vi "SW_Load_settings_to_main_tab_4.vi"(0 "Settings path in":path, 2 "Researcher name":string="Researcher", 3 "error in (no error)":errorcluster) -> (6 "Settings cluster out":T1={"Defaults"={"Default User"=0.0, "VISA Resource Name "="", "Histogram parameters"={"max"=300.0, "min"=0.0, "# bins"=10, "threshold"=8.0, "thr. type"=enum."higher accepted"}}, "Recording and saving"={"Researcher name"="", "Name prefix"="", "Data post-processing"={"Filter type"=enum."Savitzky-Golay", "Length"=31, "Order"=3}, "Stop at"=0.0, "\"Stop at\" enabled"=FALSE, "Default save folder path"=path "", "Acquisition FPS"=enum."Max"}, "Geometry"={"Sensor board size"=enum."", "Bridge swap"=FALSE, "Twisted neck"=FALSE, "Bridge H. offset"=0.0, "Bridge V. offset"=0.0, "Magnets orientation"=0.0, "Cage type"=0, "Cage parameters"={"Round"=variant(i16 0), "Square"=variant(u16 0), "Donut-maze"=variant(u16 0), "T-maze"=variant(u8 0), "Sociability-maze"=variant(u8 0)}}, "IO parameters"={"IO general config."=0, "IO 1 configuration"=0, "IO 2 configuration"=0, "IO 3 configuration"=0, "IO 4 configuration"=0, "Activate ext. RS-232"=0, "IO inversion config."=0, "Sync capability"=1}, "Conditions presets array"=[{"Enabled"=FALSE, "Name"="", "Specifier(s)"=[], "Response"={"Response type"=enum."Air puff", "TTL port"=enum."Port 1", "TTL pulse length, ms"=0.0}, "Has been set"=FALSE}, {"Enabled"=FALSE, "Name"="", "Specifier(s)"=[], "Response"={"Response type"=enum."Air puff", "TTL port"=enum."Port 1", "TTL pulse length, ms"=0.0}, "Has been set"=FALSE}, {"Enabled"=FALSE, "Name"="", "Specifier(s)"=[], "Response"={"Response type"=enum."Air puff", "TTL port"=enum."Port 1", "TTL pulse length, ms"=0.0}, "Has been set"=FALSE}, {"Enabled"=FALSE, "Name"="", "Specifier(s)"=[], "Response"={"Response type"=enum."Air puff", "TTL port"=enum."Port 1", "TTL pulse length, ms"=0.0}, "Has been set"=FALSE}, {"Enabled"=FALSE, "Name"="", "Specifier(s)"=[], "Response"={"Response type"=enum."Air puff", "TTL port"=enum."Port 1", "TTL pulse length, ms"=0.0}, "Has been set"=FALSE}, {"Enabled"=FALSE, "Name"="", "Specifier(s)"=[], "Response"={"Response type"=enum."Air puff", "TTL port"=enum."Port 1", "TTL pulse length, ms"=0.0}, "Has been set"=FALSE}, {"Enabled"=FALSE, "Name"="", "Specifier(s)"=[], "Response"={"Response type"=enum."Air puff", "TTL port"=enum."Port 1", "TTL pulse length, ms"=0.0}, "Has been set"=FALSE}, {"Enabled"=FALSE, "Name"="", "Specifier(s)"=[], "Response"={"Response type"=enum."Air puff", "TTL port"=enum."Port 1", "TTL pulse length, ms"=0.0}, "Has been set"=FALSE}, {"Enabled"=FALSE, "Name"="", "Specifier(s)"=[], "Response"={"Response type"=enum."Air puff", "TTL port"=enum."Port 1", "TTL pulse length, ms"=0.0}, "Has been set"=FALSE}, {"Enabled"=FALSE, "Name"="", "Specifier(s)"=[], "Response"={"Response type"=enum."Air puff", "TTL port"=enum."Port 1", "TTL pulse length, ms"=0.0}, "Has been set"=FALSE}, {"Enabled"=FALSE, "Name"="", "Specifier(s)"=[], "Response"={"Response type"=enum."Air puff", "TTL port"=enum."Port 1", "TTL pulse length, ms"=0.0}, "Has been set"=FALSE}, {"Enabled"=FALSE, "Name"="", "Specifier(s)"=[], "Response"={"Response type"=enum."Air puff", "TTL port"=enum."Port 1", "TTL pulse length, ms"=0.0}, "Has been set"=FALSE}, {"Enabled"=FALSE, "Name"="", "Specifier(s)"=[], "Response"={"Response type"=enum."Air puff", "TTL port"=enum."Port 1", "TTL pulse length, ms"=0.0}, "Has been set"=FALSE}, {"Enabled"=FALSE, "Name"="", "Specifier(s)"=[], "Response"={"Response type"=enum."Air puff", "TTL port"=enum."Port 1", "TTL pulse length, ms"=0.0}, "Has been set"=FALSE}], "Calibration parameters"={"Timing calibration sw/hw"=1.0, "True FPS"=80.0, "True frame time, s"=80.0, "Disp. calibration info"=[]}, "Settings loaded OK"=FALSE} {"Calibration parameters"."True frame time, s" format="%.10g"; "Calibration parameters"."Disp. calibration info"."Speed, µl per ms" format="%.3g"; "Calibration parameters"."True FPS" format="%.10g"; "Calibration parameters"."Timing calibration sw/hw" format="%.10g"; "Conditions presets array"."Specifier(s)"."Validity criteria(s)"."Validity value" min=0.0 step=0.1 format="%.2g"; "Conditions presets array"."Specifier(s)"."Value" step=1.0 format="%#.2g"; "Recording and saving"."Data post-processing"."Order" min=3 max=11 step=2; "Recording and saving"."Data post-processing"."Length" min=5 max=301 step=2; "Geometry"."Cage type" items=["Round", "Square", "Donut-maze", "T-maze", "Sociability maze", ""]}, 7 "Settings file path out":path, 10 "Error Out":errorcluster)   [LabVIEW 2018, in "Tracker.lvlib"]
uses:
  Tracker.lvlib
  Controls/CTL_Settings_cluster.ctl
  Controls/CTL_Histogram_parameters.ctl
  Controls/CTL_Filter_selector.ctl
  Controls/CTL_Acquisition_speed_selector.ctl
  Controls/CTL_Segmented_plot_parameters_2.ctl
  Libraries/Cage Diagram/Typedefs/CTL_Cage_type.ctl
  Controls/CTL_Cage_all_segmentation_params_set.ctl
  Controls/CTL_IO_params_cluster.ctl
  Controls/CTL_Conditions_Array.ctl
  Controls/CTL_Conditions_Cluster.ctl
  Controls/CTL_Condition_type.ctl
  Controls/CTL_Comparison_type.ctl
  Controls/CTL_Validity_check_criteria.ctl
  Controls/CTL_Response_info.ctl
  Controls/CTL_Condition_response_type.ctl
  Controls/CTL_Reponse_port_info.ctl
  Controls/CTL_Calibration_parameters.ctl
  Controls/CTL_Dispenser_calibration_info.ctl
  Controls/CTL_Conditions_GZippped_string.ctl
  Controls/CTL_Segmented_plot_parameters_2_(round_d1).ctl
  <vilib>/Utility/sysdir.llb/System Directory Type.ctl
  <vilib>/Utility/config.llb/NI_LVConfig.lvlib
  Common_Resources.lvlib
  Controls/CTL_Conditions_All_Presets_Cluster.ctl
  Libraries/Cage Diagram/Cage Diagram.lvlib
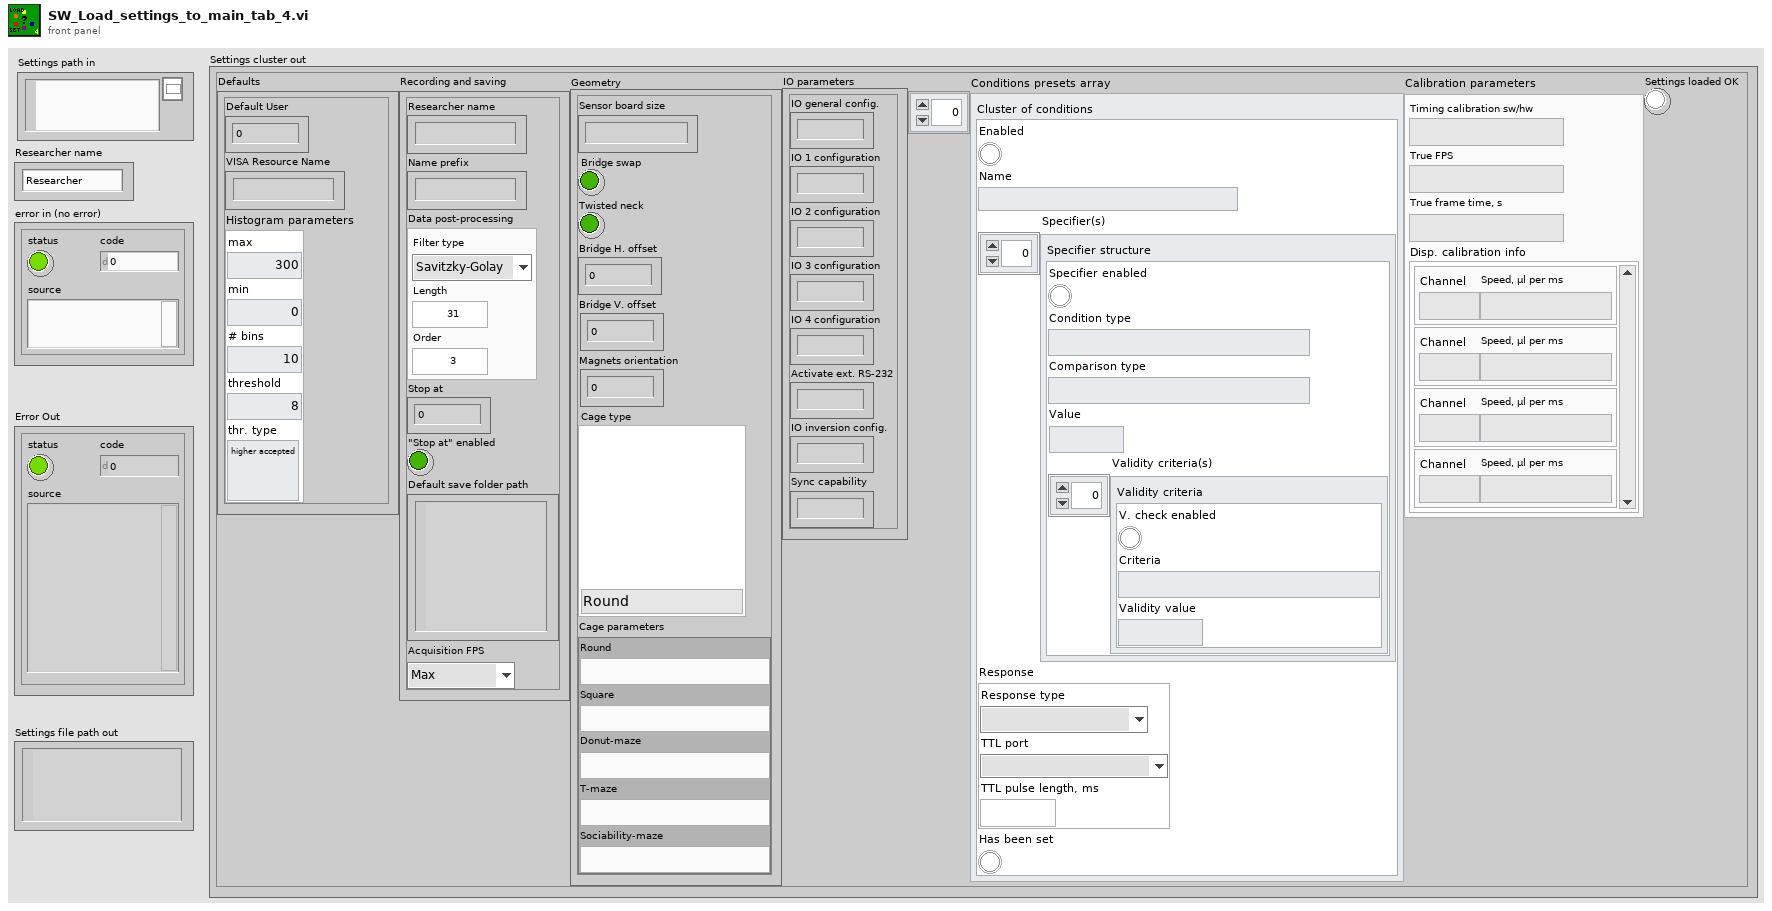
[diagram p1: front panel]
types:
  T1 = typedef "Common_Resources.lvlib/CTL_Settings_cluster.ctl" = cluster{"Defaults":cluster{"Default User":dbl, "VISA Resource Name ":string, "Histogram parameters":T2}, "Recording and saving":cluster{"Researcher name":string, "Name prefix":string, "Data post-processing":T3, "Stop at":dbl, "\"Stop at\" enabled":bool, "Default save folder path":path, "Acquisition FPS":T4}, "Geometry":T5, "IO parameters":T8, "Conditions presets array":T9, "Calibration parameters":T17, "Settings loaded OK":bool}
  T2 = typedef "Common_Resources.lvlib/CTL_Histogram_parameters.ctl" = cluster{"max":dbl, "min":dbl, "# bins":i32, "threshold":dbl, "thr. type":enum16{"higher accepted", "lower accepted"}}
  T3 = typedef "Common_Resources.lvlib/CTL_Filter_selector.ctl" = cluster{"Filter type":enum16{"None", "Savitzky-Golay"}, "Length":i32, "Order":i32}
  T4 = typedef "Common_Resources.lvlib/CTL_Acquisition_speed_selector.ctl" = enum16{"Max", "Optimal", "Eco"}
  T5 = typedef "Common_Resources.lvlib/CTL_Segmented_plot_parameters_2.ctl" = cluster{"Sensor board size":enum16{"", "Large"}, "Bridge swap":bool, "Twisted neck":bool, "Bridge H. offset":sgl, "Bridge V. offset":sgl, "Magnets orientation":sgl, "Cage type":T6, "Cage parameters":T7}
  T6 = typedef "Cage Diagram.lvlib/CTL_Cage_type.ctl" = u16
  T7 = typedef "Common_Resources.lvlib/CTL_Cage_all_segmentation_params_set.ctl" = cluster{"Round":variant, "Square":variant, "Donut-maze":variant, "T-maze":variant, "Sociability-maze":variant}
  T8 = typedef "Common_Resources.lvlib/CTL_IO_params_cluster.ctl" = cluster{"IO general config.":u16, "IO 1 configuration":u16, "IO 2 configuration":u16, "IO 3 configuration":u16, "IO 4 configuration":u16, "Activate ext. RS-232":u16, "IO inversion config.":u16, "Sync capability":u8}
  T9 = typedef "Common_Resources.lvlib/CTL_Conditions_Array.ctl" = T10[]
  T10 = typedef "Common_Resources.lvlib/CTL_Conditions_Cluster.ctl" = cluster{"Enabled":bool, "Name":string, "Specifier(s)":cluster{"Specifier enabled":bool, "Condition type":T11, "Comparison type":T12, "Value":dbl, "Validity criteria(s)":cluster{"V. check enabled":bool, "Criteria":T13, "Validity value":dbl}[]}[], "Response":T14, "Has been set":bool}
  T11 = typedef "Common_Resources.lvlib/CTL_Condition_type.ctl" = enum16{"Speed", "Zone", "Angle to wall"}
  T12 = typedef "Common_Resources.lvlib/CTL_Comparison_type.ctl" = enum16{"Less", "Less or Equal", "Equal", "Greater or Equal", "Greater", "Not Equal"}
  T13 = typedef "Common_Resources.lvlib/CTL_Validity_check_criteria.ctl" = enum16{"Running bout (seconds)", "Running bout (meters)"}
  T14 = typedef "Common_Resources.lvlib/CTL_Response_info.ctl" = cluster{"Response type":T15, "TTL port":T16, "TTL pulse length, ms":dbl}
  T15 = typedef "Common_Resources.lvlib/CTL_Condition_response_type.ctl" = enum16{"None", "Air puff", "Liquid reward", "TTL pulse", "TTL pulse (ubr)", "TTL signal"}
  T16 = typedef "Common_Resources.lvlib/CTL_Reponse_port_info.ctl" = enum16{"Port 1", "Port 2", "Port 3", "Port 4"}
  T17 = typedef "Common_Resources.lvlib/CTL_Calibration_parameters.ctl" = cluster{"Timing calibration sw/hw":dbl, "True FPS":dbl, "True frame time, s":dbl, "Disp. calibration info":T18}
  T18 = typedef "Common_Resources.lvlib/CTL_Dispenser_calibration_info.ctl" = cluster{"Channel":u8, "Speed, µl per ms":dbl}[]
  T19 = typedef "Common_Resources.lvlib/CTL_Segmented_plot_parameters_2_(round_d1).ctl" = cluster{"Cage diameter, mm":u16, "Starting angle BORDER":i16, "Starting angle MIDFIELD":i16, "Radius, mm MIDFIELD":u16, "Radius, mm CENTER":u16, "N segments BORDER":u8, "N segments MIDFIELD":u8, "R-gap, mm":sgl}
  T20 = typedef "Common_Resources.lvlib/CTL_Conditions_GZippped_string.ctl" = cluster{"GZipped XML string":string}
  T21 = typedef "Common_Resources.lvlib/CTL_Conditions_All_Presets_Cluster.ctl" = cluster{"[0]":string, "[1]":string, "[2]":string, "[3]":string, "[4]":string, "[5]":string, "[6]":string, "[7]":string, "[8]":string}
  T22 = typedef "NI_LVConfig.lvlib/Config Data RefNum.ctl" = refnum<k1>
  T23 = cluster{"Default User":dbl, "VISA Resource Name ":string, "Histogram parameters":T2}
  T24 = cluster{"Researcher name":string, "Name prefix":string, "Data post-processing":T3, "Stop at":dbl, "\"Stop at\" enabled":bool, "Default save folder path":path, "Acquisition FPS":T4}
  T25 = typedef "System Directory Type.ctl" = i32
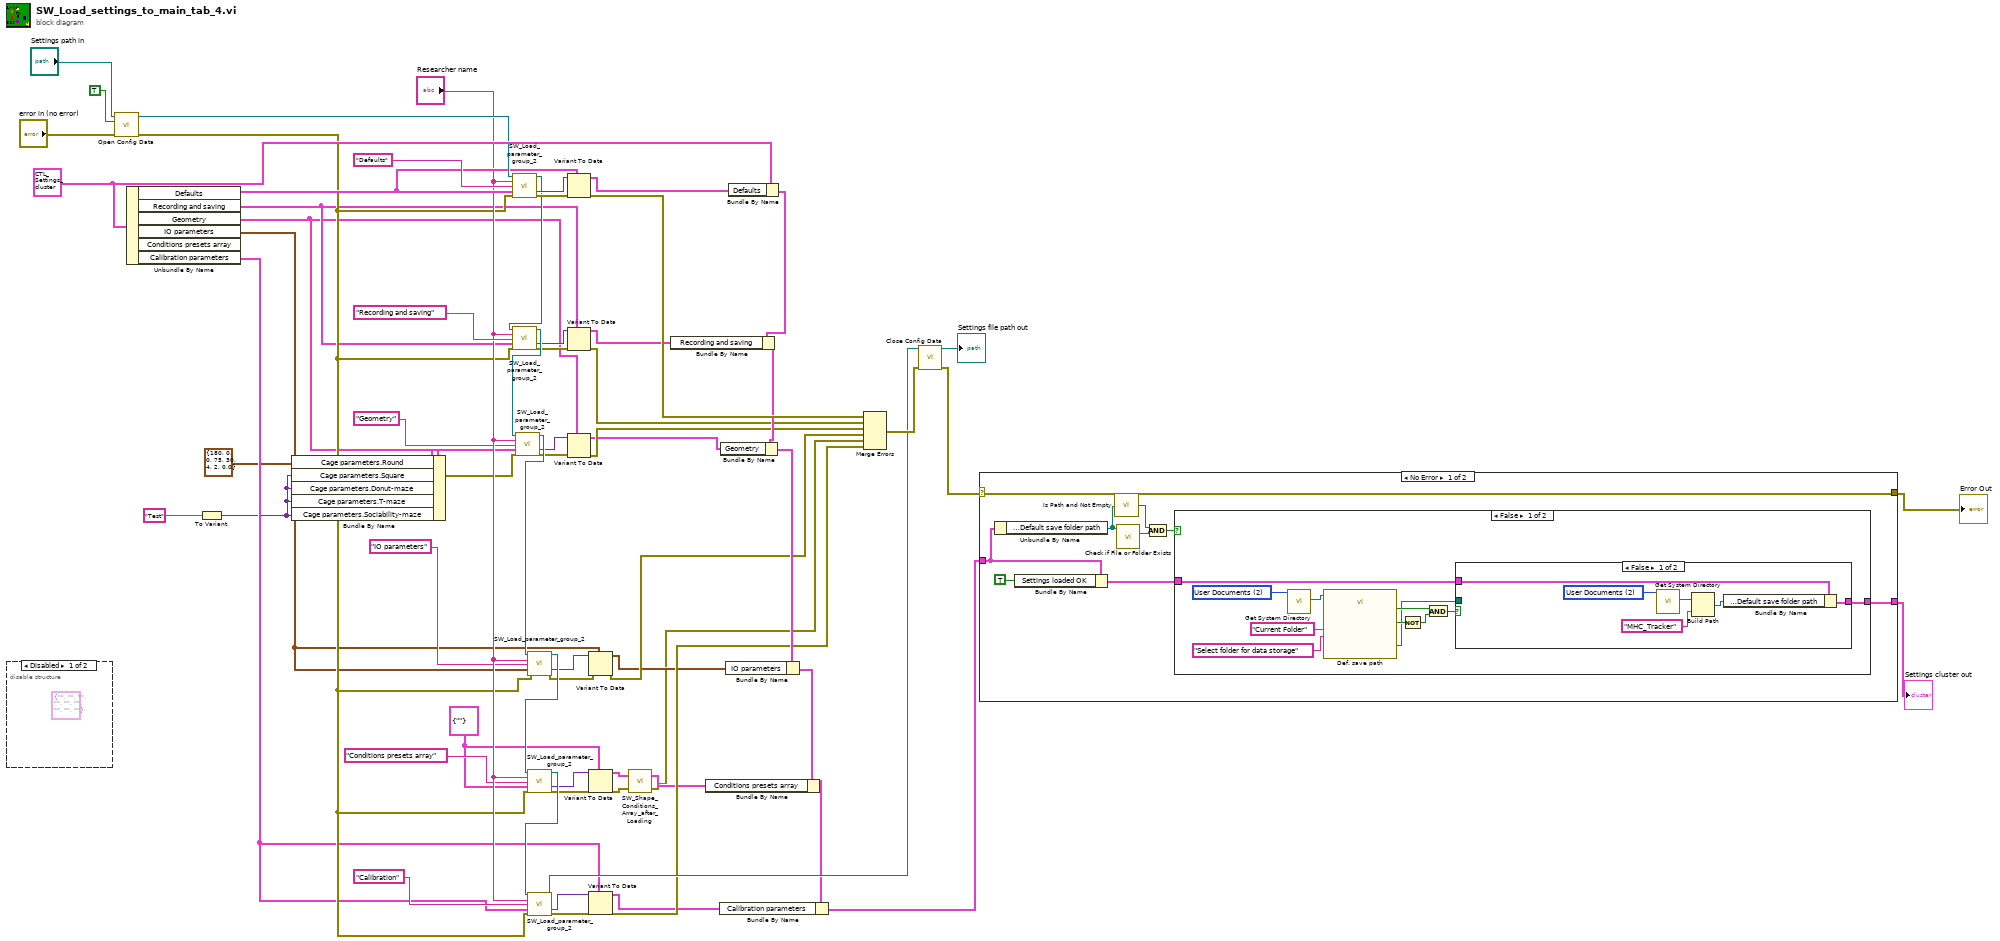
[diagram p0: block diagram]
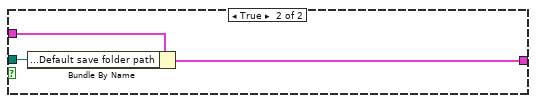
[diagram p3: hidden frame]
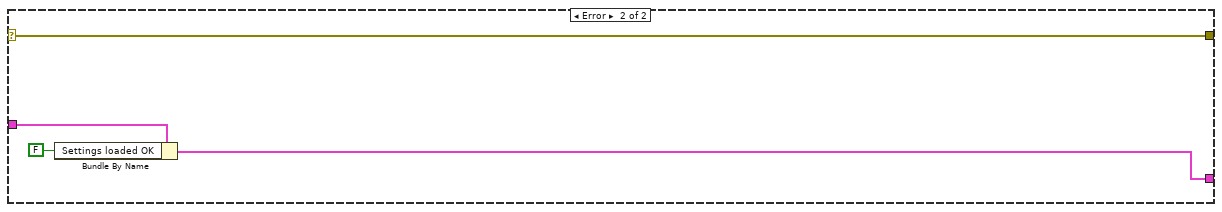
[diagram p5: hidden frame]
diagram:
  w7 = T20 {"GZipped XML string"=""} ("Conditions presets GZipped in")
  w63 = T1 {"Defaults"={"Default User"=0.0, "VISA Resource Name "="", "Histogram parameters"={"max"=300.0, "min"=0.0, "# bins"=10, "threshold"=8.0, "thr. type"=enum."higher accepted"}}, "Recording and saving"={"Researcher name"="Researcher", "Name prefix"="Track", "Data post-processing"={"Filter type"=enum."Savitzky-Golay", "Length"=31, "Order"=3}, "Stop at"=0.0, "\"Stop at\" enabled"=FALSE, "Default save folder path"=path "", "Acquisition FPS"=enum."Max"}, "Geometry"={"Sensor board size"=enum."", "Bridge swap"=FALSE, "Twisted neck"=FALSE, "Bridge H. offset"=0.0, "Bridge V. offset"=0.0, "Magnets orientation"=180.0, "Cage type"=0, "Cage parameters"={"Round"=variant(i16 0), "Square"=variant(u16 30), "Donut-maze"=variant(u16 75), "T-maze"=variant(u8 2), "Sociability-maze"=variant(u8 4)}}, "IO parameters"={"IO general config."=12, "IO 1 configuration"=1, "IO 2 configuration"=1, "IO 3 configuration"=0, "IO 4 configuration"=0, "Activate ext. RS-232"=0, "IO inversion config."=0, "Sync capability"=1}, "Conditions presets array"=[{"Enabled"=FALSE, "Name"="", "Specifier(s)"=[], "Response"={"Response type"=enum."Air puff", "TTL port"=enum."Port 1", "TTL pulse length, ms"=0.0}, "Has been set"=FALSE}, {"Enabled"=FALSE, "Name"="", "Specifier(s)"=[], "Response"={"Response type"=enum."Air puff", "TTL port"=enum."Port 1", "TTL pulse length, ms"=0.0}, "Has been set"=FALSE}, {"Enabled"=FALSE, "Name"="", "Specifier(s)"=[], "Response"={"Response type"=enum."Air puff", "TTL port"=enum."Port 1", "TTL pulse length, ms"=0.0}, "Has been set"=FALSE}, {"Enabled"=FALSE, "Name"="", "Specifier(s)"=[], "Response"={"Response type"=enum."Air puff", "TTL port"=enum."Port 1", "TTL pulse length, ms"=0.0}, "Has been set"=FALSE}, {"Enabled"=FALSE, "Name"="", "Specifier(s)"=[], "Response"={"Response type"=enum."Air puff", "TTL port"=enum."Port 1", "TTL pulse length, ms"=0.0}, "Has been set"=FALSE}, {"Enabled"=FALSE, "Name"="", "Specifier(s)"=[], "Response"={"Response type"=enum."Air puff", "TTL port"=enum."Port 1", "TTL pulse length, ms"=0.0}, "Has been set"=FALSE}, {"Enabled"=FALSE, "Name"="", "Specifier(s)"=[], "Response"={"Response type"=enum."Air puff", "TTL port"=enum."Port 1", "TTL pulse length, ms"=0.0}, "Has been set"=FALSE}, {"Enabled"=FALSE, "Name"="", "Specifier(s)"=[], "Response"={"Response type"=enum."Air puff", "TTL port"=enum."Port 1", "TTL pulse length, ms"=0.0}, "Has been set"=FALSE}, {"Enabled"=FALSE, "Name"="", "Specifier(s)"=[], "Response"={"Response type"=enum."Air puff", "TTL port"=enum."Port 1", "TTL pulse length, ms"=0.0}, "Has been set"=FALSE}, {"Enabled"=FALSE, "Name"="", "Specifier(s)"=[], "Response"={"Response type"=enum."Air puff", "TTL port"=enum."Port 1", "TTL pulse length, ms"=0.0}, "Has been set"=FALSE}, {"Enabled"=FALSE, "Name"="", "Specifier(s)"=[], "Response"={"Response type"=enum."Air puff", "TTL port"=enum."Port 1", "TTL pulse length, ms"=0.0}, "Has been set"=FALSE}, {"Enabled"=FALSE, "Name"="", "Specifier(s)"=[], "Response"={"Response type"=enum."Air puff", "TTL port"=enum."Port 1", "TTL pulse length, ms"=0.0}, "Has been set"=FALSE}, {"Enabled"=FALSE, "Name"="", "Specifier(s)"=[], "Response"={"Response type"=enum."Air puff", "TTL port"=enum."Port 1", "TTL pulse length, ms"=0.0}, "Has been set"=FALSE}, {"Enabled"=FALSE, "Name"="", "Specifier(s)"=[], "Response"={"Response type"=enum."Air puff", "TTL port"=enum."Port 1", "TTL pulse length, ms"=0.0}, "Has been set"=FALSE}], "Calibration parameters"={"Timing calibration sw/hw"=1.0, "True FPS"=80.0, "True frame time, s"=80.0, "Disp. calibration info"=[{"Channel"=1, "Speed, µl per ms"=1.0}, {"Channel"=2, "Speed, µl per ms"=1.0}, {"Channel"=3, "Speed, µl per ms"=1.0}, {"Channel"=4, "Speed, µl per ms"=1.0}]}, "Settings loaded OK"=FALSE} ("Settings cluster")
  n1 = disable-structure shown="Disabled" {
    frame Disabled {
      (unwired) T21 {"[0]"="", "[1]"="", "[2]"="", "[3]"="", "[4]"="", "[5]"="", "[6]"="", "[7]"="", "[8]"=""} ("Condition presets prepared for saving out")
    }
    frame Enabled {
    }
  }
  n2 = call <vilib>:"Open Config Data.vi"("error in (no error)"="error in (no error)", "create file if necessary (T)"=TRUE, "configuration file path"="Settings path in") -> ("error out"=w31:errorcluster, "refnum"=w52:T22)  [unwired: 6 in, 1 out]
  n3 = Unbundle By Name(w63) -> ("Defaults"=w48:T23, "Recording and saving"=w18:T24, "Geometry"=w5:T5, "IO parameters"=w15:T8, "Calibration parameters"=w13:T17)  [unwired: 1 out]
  n4 = To Variant(anything="Test") -> (Variant=w1:variant)
  n5 = Bundle By Name(cluster=w5, "Cage parameters.Round"=T19 {"Cage diameter, mm"=180, "Starting angle BORDER"=0, "Starting angle MIDFIELD"=0, "Radius, mm MIDFIELD"=75, "Radius, mm CENTER"=30, "N segments BORDER"=4, "N segments MIDFIELD"=2, "R-gap, mm"=0.0} ("Radial segmentation parameters"), "Cage parameters.Square"=w1, "Cage parameters.Donut-maze"=w1, "Cage parameters.T-maze"=w1, "Cage parameters.Sociability-maze"=w1) -> (w4:T5)
  n6 = call "SW_Load_parameter_group_2.vi"("Settings file refnum in"=w52, "Researcher name"="Researcher name", "Parameter group (section)"="Defaults" ("Group"), "Default value data in"=w48, "error in"=w31) -> ("Settings file refnum out"=w39:T22, "Group (section) cluster data out"=w49:variant, "error out"=w51:errorcluster)  [unwired: 8 in]
  n7 = call "SW_Load_parameter_group_2.vi"("Settings file refnum in"=w39, "Researcher name"="Researcher name", "Parameter group (section)"="Recording and saving" ("Group"), "Default value data in"=w18, "error in"=w31) -> ("Settings file refnum out"=w38:T22, "Group (section) cluster data out"=w30:variant, "error out"=w32:errorcluster)  [unwired: 8 in]
  n8 = call "SW_Load_parameter_group_2.vi"("Settings file refnum in"=w38, "Researcher name"="Researcher name", "Parameter group (section)"="Geometry" ("Group"), "Default value data in"=w4, "error in"=w31) -> ("Settings file refnum out"=w37:T22, "Group (section) cluster data out"=w28:variant, "error out"=w29:errorcluster)  [unwired: 8 in]
  n9 = call "SW_Load_parameter_group_2.vi"("Settings file refnum in"=w37, "Researcher name"="Researcher name", "Parameter group (section)"="IO parameters" ("Group"), "Default value data in"=w15, "error in"=w31) -> ("Settings file refnum out"=w36:T22, "Group (section) cluster data out"=w21:variant, "error out"=w33:errorcluster)  [unwired: 8 in]
  n10 = call "SW_Load_parameter_group_2.vi"("Settings file refnum in"=w36, "Researcher name"="Researcher name", "Parameter group (section)"="Conditions presets array" ("Group"), "Default value data in"=w7, "error in"=w31) -> ("Settings file refnum out"=w35:T22, "Group (section) cluster data out"=w20:variant, "error out"=w26:errorcluster)  [unwired: 8 in]
  n11 = call "SW_Load_parameter_group_2.vi"("Settings file refnum in"=w35, "Researcher name"="Researcher name", "Parameter group (section)"="Calibration" ("Group"), "Default value data in"=w13, "error in"=w31) -> ("Settings file refnum out"=w56:T22, "Group (section) cluster data out"=w19:variant, "error out"=w27:errorcluster)  [unwired: 8 in]
  n12 = Variant To Data(error in=w51, type=w48, Variant=w49) -> (data=w47:T23, error out=w50:errorcluster)
  n13 = Variant To Data(error in=w32, type=w18, Variant=w30) -> (data=w17:T24, error out=w25:errorcluster)
  n14 = Variant To Data(error in=w29, type=w5, Variant=w28) -> (data=w16:T5, error out=w24:errorcluster)
  n15 = Variant To Data(error in=w33, type=w15, Variant=w21) -> (data=w14:T8, error out=w23:errorcluster)
  n16 = Variant To Data(error in=w26, type=w7, Variant=w20) -> (data=w10:T20, error out=w11:errorcluster)
  n17 = Variant To Data(error in=w27, type=w13, Variant=w19) -> (data=w12:T17, error out=w22:errorcluster)
  n18 = call "SW_Shape_Conditions_Array_after_Loading.vi"("error in (no error)"=w11, "Conditions presets GZipped in"=w10) -> ("error out"=w8:errorcluster, "Conditions presets array out"=w9:T9)
  n19 = Bundle By Name(cluster=w63, "Defaults"=w47) -> (w46:T1)
  n20 = Bundle By Name(cluster=w46, "Recording and saving"=w17) -> (w34:T1)
  n21 = Bundle By Name(cluster=w34, "Geometry"=w16) -> (w62:T1)
  n22 = Bundle By Name(cluster=w62, "IO parameters"=w14) -> (w61:T1)
  n23 = Bundle By Name(cluster=w61, "Conditions presets array"=w9) -> (w55:T1)
  n24 = Bundle By Name(cluster=w55, "Calibration parameters"=w12) -> (w54:T1)
  n25 = Merge Errors(w50, w25, w24, w23, w8, w22) -> (w60:errorcluster)
  n26 = call <vilib>:"Close Config Data.vi"("error in (no error)"=w60, "refnum"=w56) -> ("error out"=w59:errorcluster, "file path"=→"Settings file path out":path)  [unwired: 8 in]
  n27 = case shown="No Error" w59 {
    selector: w59 -> [w74 w98]
    tunnel: [w74 w98] -> w6
    tunnel: w54 -> [w73 w100]
    tunnel: [w67 w97] -> w58
    frame No Error {
      n28 = Unbundle By Name(w73) -> ("Recording and saving.Default save folder path"=w71:path)
      n29 = Bundle By Name(cluster=w73, "Settings loaded OK"=TRUE) -> (w68:T1)
      n30 = call <vilib>:"Is Path and Not Empty.vi"("path"=w71) -> ("Is Path and Not Empty?"=w72:bool)  [unwired: 4 in]
      n31 = call <vilib>:"Check if File or Folder Exists.vi"("path"=w71) -> ("file or folder exists?"=w70:bool)  [unwired: 8 in, 2 out]
      n32 = And(x=w72, y=w70) -> (x .and. y?=w69:bool)
      n33 = case shown="False" w69 {
        tunnel: w68 -> [w78 w96]
        tunnel: [w77 w96] -> w67
        frame False {
          w85 = T25 2 items=["User Home"=0, "User Desktop"=1, "User Documents"=2, "User Application Data"=3, "User Preferences"=4, "User Temporary"=5, "Public Documents"=6, "Public Application Data"=7, "Public Preferences"=8, "Public Cache"=13, "System Core Libraries"=9, "System Installed Libraries"=10, "Application Files"=11, "Boot Volume Root"=12] ("system directory type")
          n34 = call <vilib>:"Get System Directory.vi"("system directory type"=w85) -> ("system directory"=w86:path)  [unwired: 10 in]
          n35 = call "Def. save path"("start path"=w86, "prompt"="Select folder for data storage", "button label"="Current Folder") -> ("selected path"=w76:path, "exists"=w80:bool, "cancelled"=w82:bool)  [unwired: 9 in, 1 out]
          n36 = Not(x=w82) -> (.not. x?=w81:bool)
          n37 = And(x=w80, y=w81) -> (x .and. y?=w79:bool)
          n38 = case shown="False" w79 {
            tunnel: w78 -> [w88 w95]
            tunnel: [w87 w94] -> w77
            tunnel: w76 -> [_ w93]
            frame False {
              w91 = T25 2 items=["User Home"=0, "User Desktop"=1, "User Documents"=2, "User Application Data"=3, "User Preferences"=4, "User Temporary"=5, "Public Documents"=6, "Public Application Data"=7, "Public Preferences"=8, "Public Cache"=13, "System Core Libraries"=9, "System Installed Libraries"=10, "Application Files"=11, "Boot Volume Root"=12] ("system directory type")
              n39 = call <vilib>:"Get System Directory.vi"("system directory type"=w91) -> ("system directory"=w92:path)  [unwired: 10 in]
              n40 = Build Path(base path=w92, name or relative path="MHC_Tracker") -> (appended path=w90:path)
              n41 = Bundle By Name(cluster=w88, "Recording and saving.Default save folder path"=w90) -> (w87:T1)
            }
            frame True {
              n42 = Bundle By Name(cluster=w95, "Recording and saving.Default save folder path"=w93) -> (w94:T1)
            }
          }
        }
        frame True {
        }
      }
    }
    frame Error {
      n43 = Bundle By Name(cluster=w100, "Settings loaded OK"=FALSE) -> (w97:T1)
    }
  }
  "Settings cluster out" <- w58
  "Error Out" <- w6
